vi "Init Lidar Labview.vi"(8 "error in (no error)":errorcluster) -> (0 "error out":errorcluster)   [LabVIEW 2017]
uses:
  <instrlib>/Hokuyo URG Series/Public/Initialize-Standard.vi
  Variables/Labview lidar globals.vi
  <instrlib>/Hokuyo URG Series/Hokuyo URG Series.lvlib
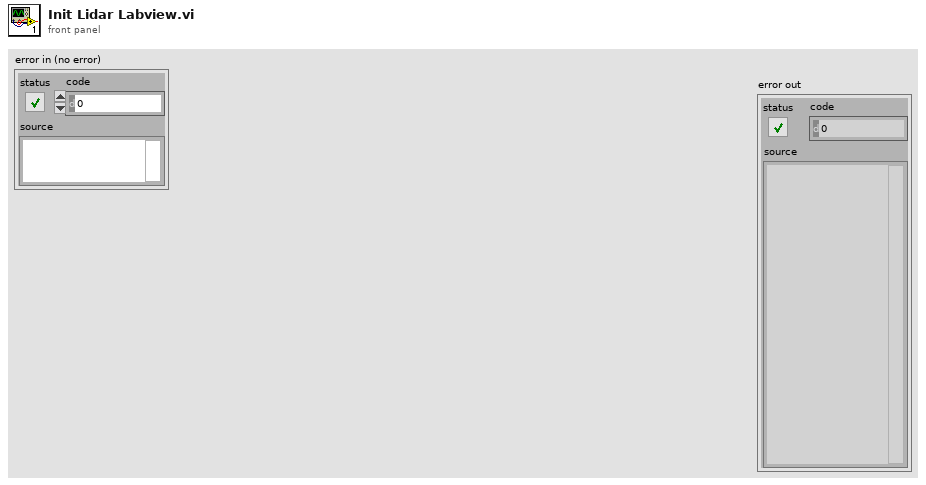
[diagram p1: front panel]
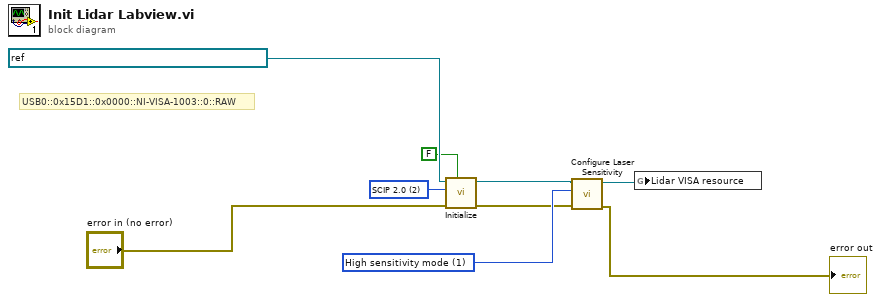
[diagram p0: block diagram]
diagram:
  w6 = u32 1 items=["Normal mode", "High sensitivity mode"] ("Sensitivity Mode (0: Normal mode)")
  w9 = u32 2 items=["Convert to Latest", "SCIP 1.1", "SCIP 2.0"] ("Protocol (2: SCIP 2.0)")
  # "USB0::0x15D1::0x0000::NI-VISA-1003::0::RAW"
  n1 = call-poly <instrlib>:"Initialize.vi"("ID Query? (Enabled)"=FALSE, "error in (no error)"="error in (no error)", "Protocol (2: SCIP 2.0)"=w9, "VISA resource name"=refnum<visa-resource-name> "USB0::0x15D1::0x0000::NI-VISA-1002::1::RAW") -> ("error out"=w5:errorcluster, "VISA resource name out"=w7:refnum<visa-resource-name>)  [unwired: 6 in]
  n2 = call <instrlib>:"Configure Laser Sensitivity.vi"("error in (no error)"=w5, "Sensitivity Mode (0: Normal mode)"=w6, "VISA resource name"=w7) -> ("error out"=→"error out":errorcluster, "VISA resource name out"=w3:refnum<visa-resource-name>)  [unwired: 7 in]
  n3 = global write "Labview lidar globals.vi" "Lidar VISA resource"(w3) -> ()
